vi "Destroy.vi"(8 "error in (no error)":errorcluster, 11 "reference in":refnum<class "Actor1_GUI_G4_4.0.0.lvclass">) -> (0 "error out":errorcluster, 3 "reference out":refnum<class "Actor1_GUI_G4_4.0.0.lvclass">)   [LabVIEW 2014, in "Actor1_GUI_G4_4.0.0.lvlib" / "Actor1_GUI_G4_4.0.0.lvclass"]
uses:
  <resource>/Framework/Providers/Open_GDS/ClassProviders/ActorFramework/4.0.0/Actor1_GUI_G4_4.0.0/Actor1_GUI_G4_4.0.0_Actor/Actor1_GUI_G4_4.0.0.lvclass
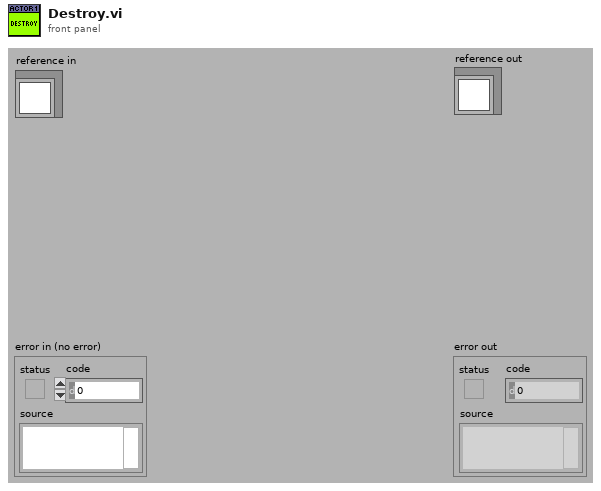
[diagram p1: front panel]
types:
  T1 = typedef "Actor1_GUI_G4_4.0.0.lvlib/Actor1_GUI_G4_4.0.0.lvclass/ObjectAttributes.ctl" = cluster{"LoopEvent":refnum<user-event>}
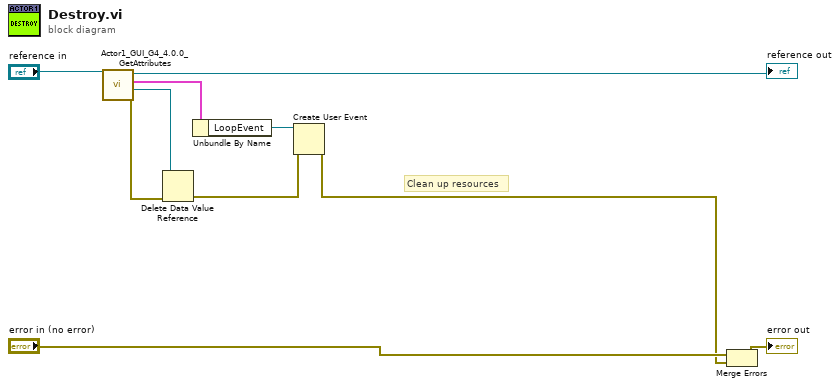
[diagram p0: block diagram]
diagram:
  # "Clean up resources"
  n1 = call <resource>:"Actor1_GUI_G4_4.0.0_GetAttributes.vi"("reference in"="reference in") -> ("error out"=w7:errorcluster, "DataRef"=w6:refnum<data-value>, "Data"=w5:T1, "reference out"=→"reference out":refnum<class "Actor1_GUI_G4_4.0.0.lvclass">)  [unwired: 7 in]
  n2 = Delete Data Value Reference(data value reference=w6, error in=w7) -> (error out=w2:errorcluster)  [unwired: 1 out]
  n3 = Unbundle By Name(w5) -> ("LoopEvent"=w3:refnum<user-event>)
  n4 = Create User Event(user event datatype=w3, error in=w2) -> (error out=w1:errorcluster)  [unwired: 1 out]
  n5 = Merge Errors("error in (no error)", w1) -> (→"error out":errorcluster)
